vi "Sweep_File_Name_String.vi"(8 "String":string, 9 "Stop":i32, 10 "Start":i32) -> (2 "Output string":string)   [LabVIEW 2022 SP3]
panel:
  out "StopStr":string
  out "StartString":string
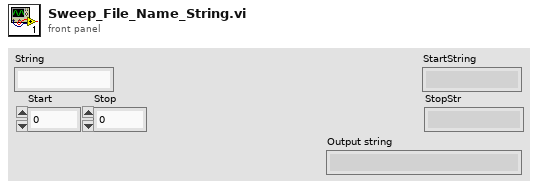
[diagram p1: front panel]
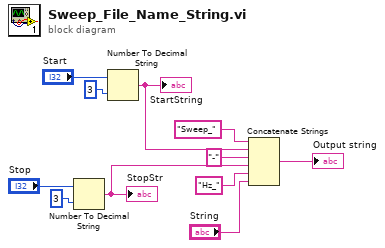
[diagram p0: block diagram]
diagram:
  n1 = Number To Decimal String(number="Stop", width (-)=i16 3) -> (decimal integer string=w6:string)
  "StopStr" <- w6
  n2 = Number To Decimal String(number="Start", width (-)=i16 3) -> (decimal integer string=w2:string)
  "StartString" <- w2
  n3 = Concatenate Strings("Sweep_" ("string"), w2, "-" ("string"), w6, "Hz_" ("string"), "String") -> (→"Output string":string)
